vi "CarDisplay(Main).vi"() -> ()   [LabVIEW 2014]
uses:
  States(Typedef).ctl
  <vilib>/MakerHub/LINX/LMH-LINX.lvlib
panel:
  in  "Need a hand?":bool
  out "Breathalyzer Graph":cluster{dbl, dbl, "Array of Values":dbl[]}(graph)
  out "Car can start?":bool
  in  "Stop Button":bool
  out "Messages":string
  out "Breathalyzer Output Value":dbl
  in  "Begin Test":bool
  # "Safe Streets Driving Interface"
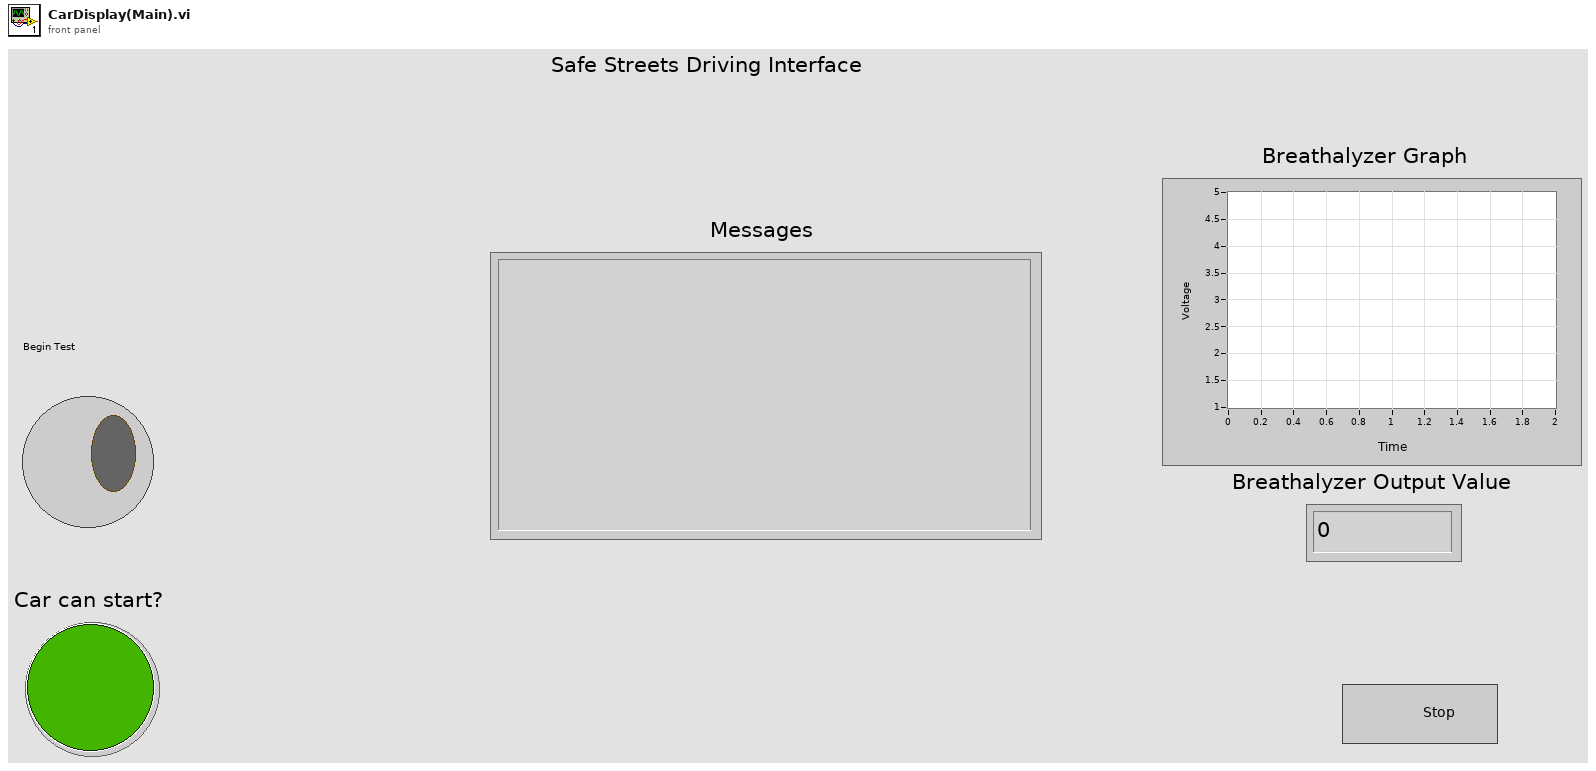
[diagram p1: front panel]
types:
  T1 = enum8{"Enabled", "Disabled", "Disabled and Grayed Out"}
  T2 = typedef "States(Typedef).ctl" = enum16{"Locked", "Breathalyze", "Unlocked", "Failed"}
  T3 = typedef "LMH-LINX.lvlib/LINX Ref.ctl" = cluster{"Platform":T4, "Interface":T5, "LINX Device Config":T6}
  T4 = typedef "LMH-LINX.lvlib/Platform.ctl" = enum16{"LINX", "myRIO"}
  T5 = typedef "LMH-LINX.lvlib/Interface.ctl" = enum16{"Serial", "TCP"}
  T6 = typedef "LMH-LINX.lvlib/Device.lvlib/LINX Device Config.ctl" = cluster{"Interface":T5, "COM Port":refnum<visa-resource-name>, "TCP Configuration":T7, "Device Family":u8, "Device ID":u8, "Device Name":string, "TCP Ref":refnum<k5>, "Channels":T8}
  T7 = typedef "LMH-LINX.lvlib/Device.lvlib/TCP Config.ctl" = cluster{"IP Address":string, "Port":u16}
  T8 = typedef "LMH-LINX.lvlib/Channels.ctl" = cluster{"DI":u8[], "DO":u8[], "AI":u8[], "AO":u8[], "PWM":u8[], "QE":u8[], "UART":u8[], "I2C 2":u8[], "SPI":u8[], "CAN":u8[], "Servo":u8[], "AI Ref (V)":dbl, "AO Ref (V)":dbl, "AO Resolution (Bits)":u8}
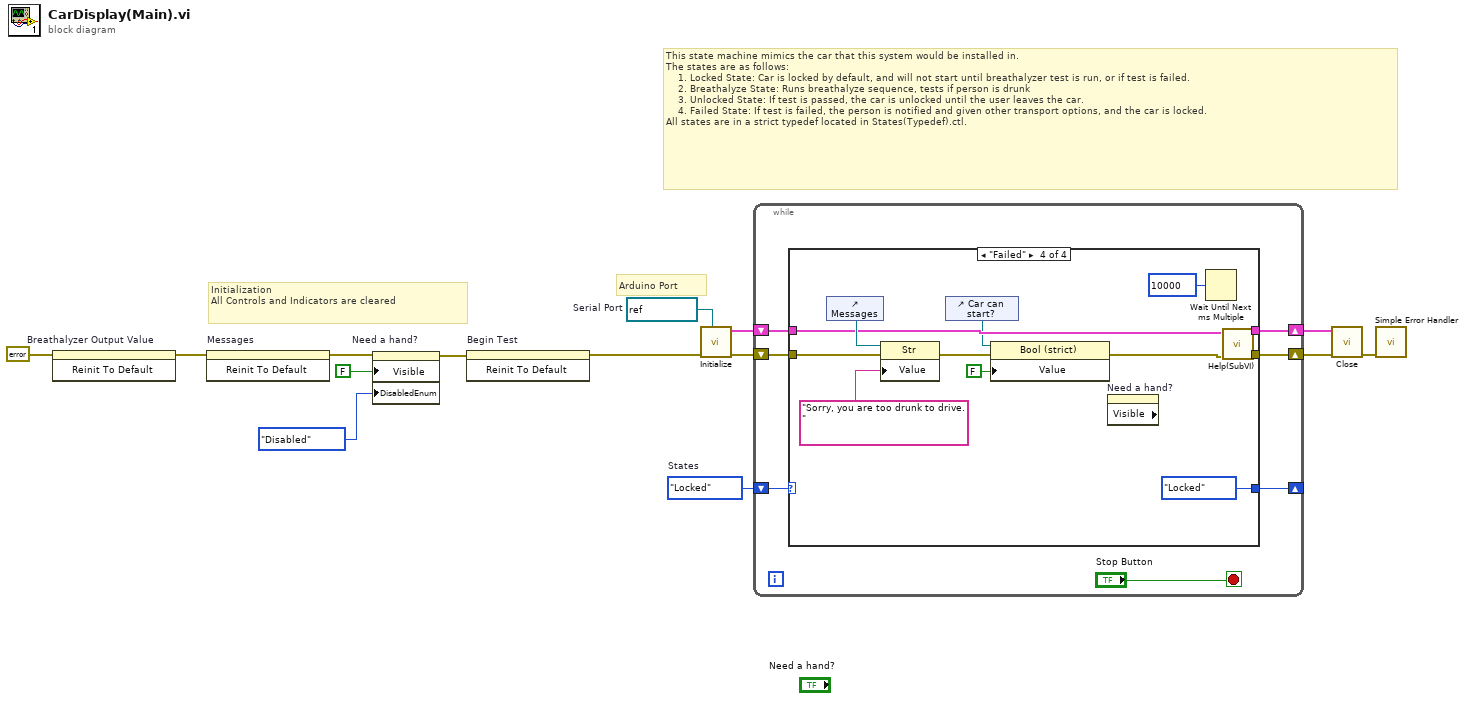
[diagram p0: block diagram]
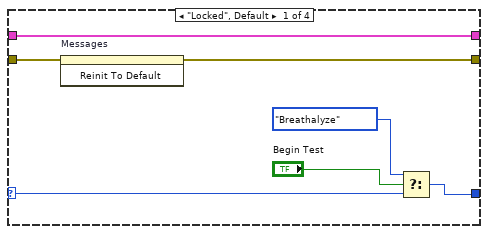
[diagram p2: hidden frame]
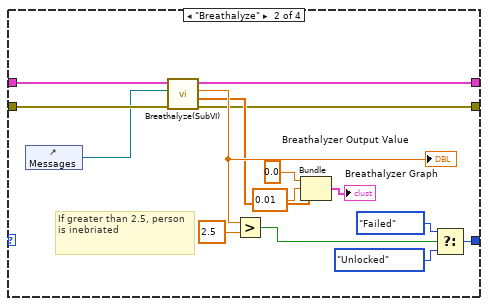
[diagram p3: hidden frame]
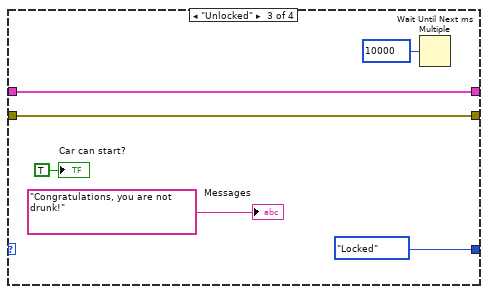
[diagram p4: hidden frame]
diagram:
  w11 = States(Typedef)."Locked"  # States
  w14 = refnum<visa-resource-name> "COM3"  # Serial Port
  # "This state machine mimics the car that this system would be installed in.\nThe states are as follows:\n    1. Locked State: Car is locked by default, and will not start until breathalyzer test is run, or if test is failed.\n    2. Breathalyze State: Runs breathalyze sequence, tests if person is drunk\n    3. Unlocked State: If test is passed, the car is unlocked until the user leaves the car.\n    4. Failed State: If test is failed, the person is notified and given other transport options, and the car is locked.\nAll states are in a strict typedef located in States(Typedef).ctl."
  # "Initialization\nAll Controls and Indicators are cleared"
  # "Arduino Port"
  n1 = invoke on="Breathalyzer Output Value" class="DigNum (strict)" method="Reinit To Default"(error in=errorcluster {"status"=FALSE, "code"=0, "source"=""} ("Error In")) -> (error out=w6:errorcluster)  [unwired: 2 in, 2 out]
  n2 = invoke on="Messages" class="Str" method="Reinit To Default"(error in=w6) -> (error out=w4:errorcluster)  [unwired: 2 in, 2 out]
  n3 = property on="Need a hand?" class="Bool"(error in=w4, "Visible"=FALSE, "DisabledEnum"=T1."Disabled" ("Disabled")) -> (error out=w3:errorcluster)  [unwired: 1 in, 1 out]
  n4 = invoke on="Begin Test" class="Bool" method="Reinit To Default"(error in=w3) -> (error out=w7:errorcluster)  [unwired: 2 in, 2 out]
  n5 = call <vilib>:"Initialize.vi"("Serial Port"=w14, "Error In"=w7) -> ("Error Out"=w13:errorcluster, "LINX Ref"=w12:T3)  [unwired: 7 in, 1 out]
  n6 = while {
    shift-right: [w18] -> _
    shift-left: w11 -> [w21]
    shift-right: [w17] -> w9
    shift-left: w13 -> [w20]
    shift-right: [w15] -> w10
    shift-left: w12 -> [w19]
    stop <- "Stop Button" stop-if-true
    n7 = case shown="\"Failed\"" w21 {
      selector: w21 -> [w27 _ _ _]
      tunnel: w20 -> [w23 w43 w49 w56]
      tunnel: w19 -> [w24 w42 w48 w52]
      tunnel: [w25 w38 States(Typedef)."Locked" ("t") States(Typedef)."Locked" ("States")] -> w18
      tunnel: [w22 w29 w49 w53] -> w17
      tunnel: [w24 w30 w48 w54] -> w15
      frame "Locked", Default {
        n8 = invoke on="Messages" class="Str" method="Reinit To Default"(error in=w23) -> (error out=w22:errorcluster)  [unwired: 2 in, 2 out]
        n9 = Select(t=States(Typedef)."Breathalyze", s="Begin Test", f=w27) -> (s? t:f=w25:T2)
      }
      frame "Breathalyze" {
        # "If greater than 2.5, person is inebriated"
        n10 = control-ref of="Messages"() -> (w41:refnum<vi>)
        n11 = call "Breathalyze(SubVI).vi"("error in (no error)"=w43, "Str Refnum"=w41, "LINX Ref"=w42) -> ("error out"=w29:errorcluster, "Array of Values"=w32:dbl[], "Average of array"=w40:dbl, "LINX Resource"=w30:T3)  [unwired: 5 in]
        "Breathalyzer Output Value" <- w40
        n12 = Greater?(x=w40, y=2.5) -> (0:w37:bool)
        n13 = Bundle(0.0, 0.01, "Array of Values"=w32) -> (→"Breathalyzer Graph":cluster{dbl, dbl, "Array of Values":dbl[]})  [unwired: 1 in]
        n14 = Select(t=States(Typedef)."Failed", s=w37, f=States(Typedef)."Unlocked") -> (s? t:f=w38:T2)
      }
      frame "Unlocked" {
        n15 = Wait Until Next ms Multiple(millisecond multiple=u32 10000) -> ()  [unwired: 1 out]
        "Messages" <- "Congratulations, you are not drunk!" ("Value")
        "Car can start?" <- TRUE ("Car can start?")
      }
      frame "Failed" {
        n16 = control-ref of="Messages"() -> (w59:refnum<vi>)
        n17 = property class="Str"(reference=w59, error in=w56, "Value"="Sorry, you are too drunk to drive.") -> (error out=w55:errorcluster)  [unwired: 1 out]
        n18 = control-ref of="Car can start?"() -> (w51:refnum<vi>)
        n19 = property class="Bool (strict)"(reference=w51, error in=w55, "Value"=FALSE) -> (error out=w50:errorcluster)  [unwired: 1 out]
        n20 = property on="Need a hand?" class="Bool" props=["Visible"]() -> ()  [unwired: 2 in, 3 out]
        n21 = Wait Until Next ms Multiple(millisecond multiple=u32 10000) -> ()  [unwired: 1 out]
        n22 = call "Help(SubVI).vi"("error in (no error)"=w50, "LINX Ref"=w52) -> ("Error Out"=w53:errorcluster, "LINX Resource"=w54:T3)  [unwired: 8 in]
      }
    }
  }
  n23 = call <vilib>:"Close.vi"("Error In"=w9, "LINX Resource"=w10) -> ("Error Out"=w8:errorcluster)  [unwired: 8 in, 1 out]
  n24 = call <vilib>:"Simple Error Handler.vi"("error in (no error)"=w8) -> ()  [unwired: 4 in, 5 out]
